vi "Open Rx Session.vi"(8 "error in (no error)":errorcluster, 11 "CAN in":refnum<class "CAN.lvclass">) -> (0 "error out":errorcluster, 3 "CAN out":refnum<class "CAN.lvclass">)   [LabVIEW 2019, in "CAN.lvclass"]
uses:
  CAN.lvclass
  CAN.lvclass/CAN.ctl
  <vilib>/xnet/xnet.llb/XNET Create Session (Signal Input Single-point).vi
  <resource>/objmgr/xnet.rc
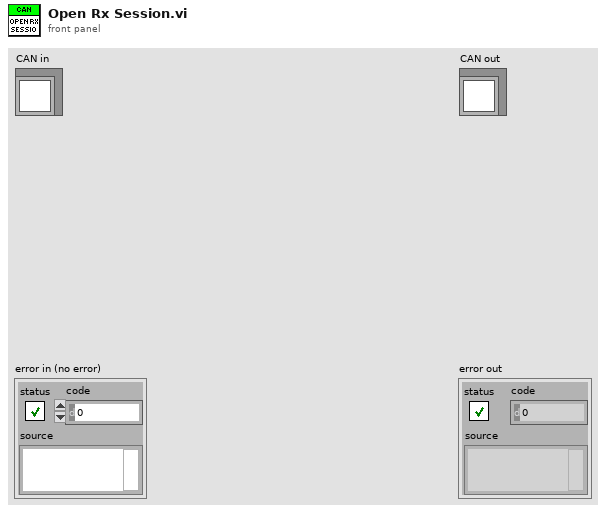
[diagram p1: front panel]
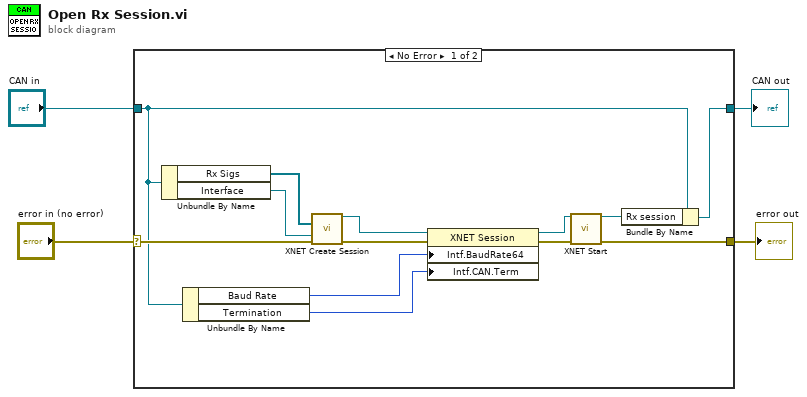
[diagram p0: block diagram]
diagram:
  n1 = case shown="No Error" "error in (no error)" {
    selector: "error in (no error)" -> [w12 w19]
    tunnel: [w10 w19] -> w3
    tunnel: [w8 w18] -> w1
    tunnel: "CAN in" -> [w7 w18]
    frame No Error {
      n2 = Unbundle By Name(w7) -> ("Rx Sigs"=w13:refnum<k21>[], "Interface"=w11:refnum<k21>)
      n3 = Unbundle By Name(w7) -> ("Baud Rate"=w6:u64, "Termination"=w5:u32)
      n4 = call-poly <vilib>:"XNET Create Session.vi"("signal list"=w13, "interface"=w11, "error in (no error)"=w12) -> ("session out"=w15:refnum<k21>, "error out"=w17:errorcluster)  [unwired: 11 out]
      n5 = property class="XNET Session"(reference=w15, error in=w17, "Intf.BaudRate64"=w6, "Intf.CAN.Term"=w5) -> (reference out=w16:refnum<k21>, error out=w14:errorcluster)
      n6 = call <vilib>:"XNET Start.vi"("session in"=w16, "error in (no error)"=w14) -> ("session out"=w9:refnum<k21>, "error out"=w10:errorcluster)  [unwired: 12 in]
      n7 = Bundle By Name(cluster=w7, "Rx session"=w9) -> (w8:refnum<class "CAN.lvclass">)
    }
    frame Error {
    }
  }
  "error out" <- w3
  "CAN out" <- w1
